vi "test build internal string.vi"() -> ()   [LabVIEW 2014]
uses:
  user.lib/_NEVSTOP/Communicable State Machine(CSM)/_Support/Typedef/_CSM_Response Source Message.ctl
  user.lib/_NEVSTOP/Communicable State Machine(CSM)/AdvanceAPI/CSM - Convert Error to Argument.vi
  user.lib/_NEVSTOP/Communicable State Machine(CSM)/Communicable State Machine.lvlib
panel:
  out "State with Arguments 2":string
  out "State with Arguments":string
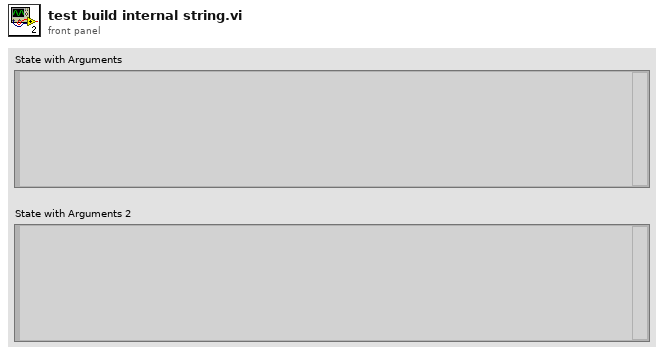
[diagram p1: front panel]
types:
  T1 = typedef "Communicable State Machine.lvlib/_CSM_Response Source Message.ctl" = cluster{"‘State":string, "’Arguments":string, "’Error":errorcluster}
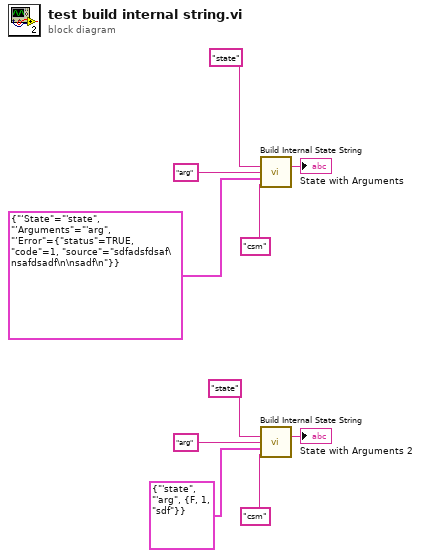
[diagram p0: block diagram]
diagram:
  n1 = call "Build Internal State String.vi"("State"="state", "Arguments (\"\")"="arg" ("Arguments (\"\")"), ">> Response Source Message >>"=T1 {"‘State"="'state", "’Arguments"="'arg", "’Error"={"status"=TRUE, "code"=1, "source"="sdfadsfdsaf\nsafdsadf\n\nsadf\n"}}, "Source (\"\")"="csm" ("Source (\"\")")) -> ("State with Arguments"=→"State with Arguments":string)  [unwired: 11 in]
  n2 = call "Build Internal State String.vi"("State"="state", "Arguments (\"\")"="arg" ("Arguments (\"\")"), ">> Response Source Message >>"=T1 {"‘State"="'state", "’Arguments"="'arg", "’Error"={"status"=FALSE, "code"=1, "source"="sdf"}}, "Source (\"\")"="csm" ("Source (\"\")")) -> ("State with Arguments"=→"State with Arguments 2":string)  [unwired: 11 in]
